vi "Configure Sample Rate Coupling.vi"(0 "VISA resource name":refnum<visa-resource-name>, 1 "Couple Ratio (1)":dbl=1.0, 2 "Couple Mode (1: Ratio)":i32(ring)=1 items=["Offset", "Ratio"], 5 "Channel (1: 1)":i32(ring)=1 items=["1"=1, "2"=2], 7 "Enable Couple(T: Enable)":bool=TRUE, 11 "error in (no error)":errorcluster, 12 "Couple Offset (0 Sa/s)":dbl) -> (4 "VISA resource name out":refnum<visa-resource-name>, 15 "error out":errorcluster)   [LabVIEW 2023, in "Keysight-33500B.lvlib"]
doc: "Configures sample rate coupling between channels. \n\n<b>Note</b>:\n(1) Both channels must be configured to Arbitraty waveform in order to enable sample rate coupling. \n(2) This VI is only valid on a 2-channel instrument."
uses:
  Keysight-33500B.lvlib
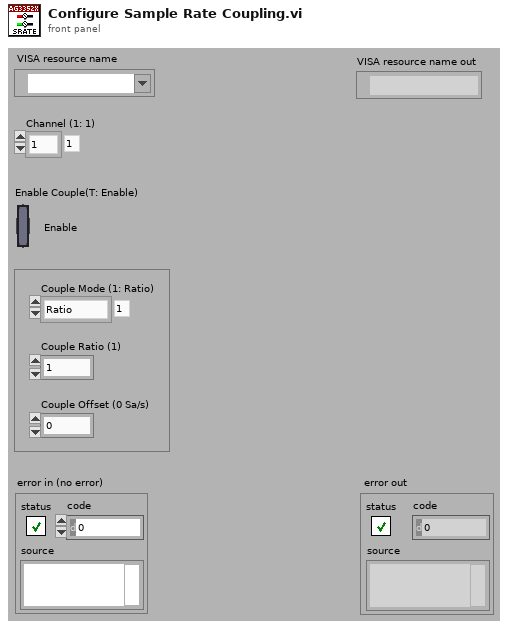
[diagram p1: front panel]
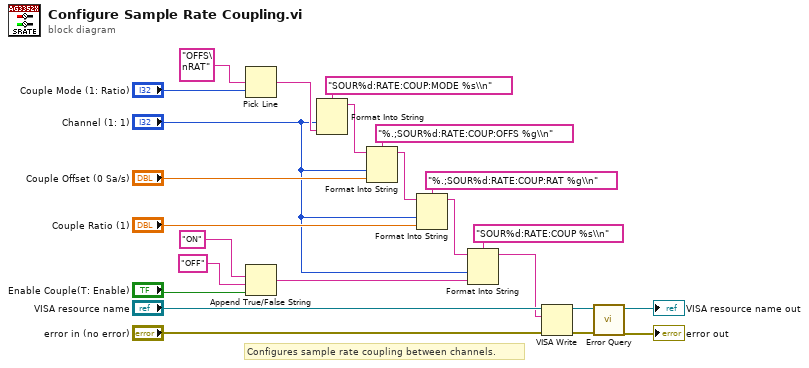
[diagram p0: block diagram]
diagram:
  # "Configures sample rate coupling between channels."
  n1 = Pick Line(multi-line string="OFFS\nRAT", line index="Couple Mode (1: Ratio)") -> (output string=w4:string)  [unwired: 1 out]
  n2 = Append True/False String(1:"Enable Couple(T: Enable)", 2:"OFF", 3:"ON") -> (0:w13:string)  [unwired: 1 out]
  n3 = Format Into String(format string="SOUR%d:RATE:COUP:MODE %s\\n", "Channel (1: 1)", w4) -> (resulting string=w23:string)  [unwired: 2 in, 1 out]
  n4 = Format Into String(format string="%.;SOUR%d:RATE:COUP:OFFS %g\\n", initial string=w23, "Channel (1: 1)", "Couple Offset (0 Sa/s)") -> (resulting string=w2:string)  [unwired: 1 in, 1 out]
  n5 = Format Into String(format string="%.;SOUR%d:RATE:COUP:RAT %g\\n", initial string=w2, "Channel (1: 1)", "Couple Ratio (1)") -> (resulting string=w15:string)  [unwired: 1 in, 1 out]
  n6 = Format Into String(format string="SOUR%d:RATE:COUP %s\\n", initial string=w15, "Channel (1: 1)", w13) -> (resulting string=w1:string)  [unwired: 1 in, 1 out]
  n7 = VISA Write(VISA resource name="VISA resource name", write buffer=w1, error in (no error)="error in (no error)") -> (VISA resource name out=w10:refnum<visa-resource-name>, error out=w9:errorcluster)  [unwired: 1 out]
  n8 = call "Error Query.vi"("error in (no error)"=w9, "VISA resource name"=w10) -> ("error out"=→"error out":errorcluster, "VISA resource name out"=→"VISA resource name out":refnum<visa-resource-name>)  [unwired: 8 out]
